vi "Sonde Single Measurement Subvi.vi"(0 "VISAResourceName in":refnum<vi>, 1 "Time Array":dbl[](array[numeric]), 2 "Cumulative Sonde Data":dbl[][](array[numeric]), 3 "Previous time":dbl, 5 "Sonde Data Display":refnum<vi>, 7 "Sonde Graph in":refnum<vi>, 9 "Temp Graph 3":refnum<vi>, 11 "error in (no error)":errorcluster, 12 "Row Cluster Input":T1={"Head\nPressure"=0.0, "Depth"=0.0, "comment "="", "Aux1"=0.0, "Aux2"=0.0, "Aux3\\EC"=0.0, "Sonde Data Cluster"={"Specific\nCond (uS)"=2.0, "Dissolved\nOxygen mg/L"=3.0, "pH"=4.0, "ORP"=5.0, "Temp (deg C)"=26.0, "Salinity"=7.0, "Dissolved\nOxygen (%)"=0.0}, "Cumulative\nVolume (ml)"=100.0} {"Cumulative\nVolume (ml)" format="%#_4g"; "Sonde Data Cluster"."Dissolved\nOxygen (%)" format="%_3g"; "Sonde Data Cluster"."Salinity" format="%_2g"; "Sonde Data Cluster"."Temp (deg C)" format="%_4g"; "Sonde Data Cluster"."ORP" format="%_4g"; "Sonde Data Cluster"."pH" format="%_4g"; "Sonde Data Cluster"."Dissolved\nOxygen mg/L" format="%_4g"; "Sonde Data Cluster"."Specific\nCond (uS)" format="%#_4g"}, 13 "reference 5":refnum<vi>) -> (4 "seconds since 1Jan1904":timestamp, 6 "Cumulative Sonde \nData Out":dbl[][](array[numeric]), 8 "Sample Sheet Data Row Cluster out":T1 {"Cumulative\nVolume (ml)" format="%#_4g"; "Sonde Data Cluster"."Dissolved\nOxygen (%)" format="%_3g"; "Sonde Data Cluster"."Salinity" format="%_2g"; "Sonde Data Cluster"."Temp (deg C)" format="%_4g"; "Sonde Data Cluster"."ORP" format="%_4g"; "Sonde Data Cluster"."pH" format="%_4g"; "Sonde Data Cluster"."Dissolved\nOxygen mg/L" format="%_4g"; "Sonde Data Cluster"."Specific\nCond (uS)" format="%#_4g"}, 10 "output cluster":T2 caption="Cluster" {"Dissolved\nOxygen (%)" format="%_3g"; "Salinity" format="%_2g"; "Temp (deg C)" format="%_4g"; "ORP" format="%_4g"; "pH" format="%_3g"; "Dissolved\nOxygen mg/L" format="%_4g"; "Specific\nCond (uS)" format="%#_4g"}, 14 "time array out":dbl[](array[numeric]), 15 "error out":errorcluster)   [LabVIEW 2016]
uses:
  activeXtest/activeXtest 2015 Folder/sonde cluster.ctl
  activeXtest/activeXtest 2015 Folder/sample data row cluster.ctl
panel:
  in  "Manual Entry Quanta Sonde Com Port":refnum<visa-resource-name>="COM12"
  out "error out 2":errorcluster
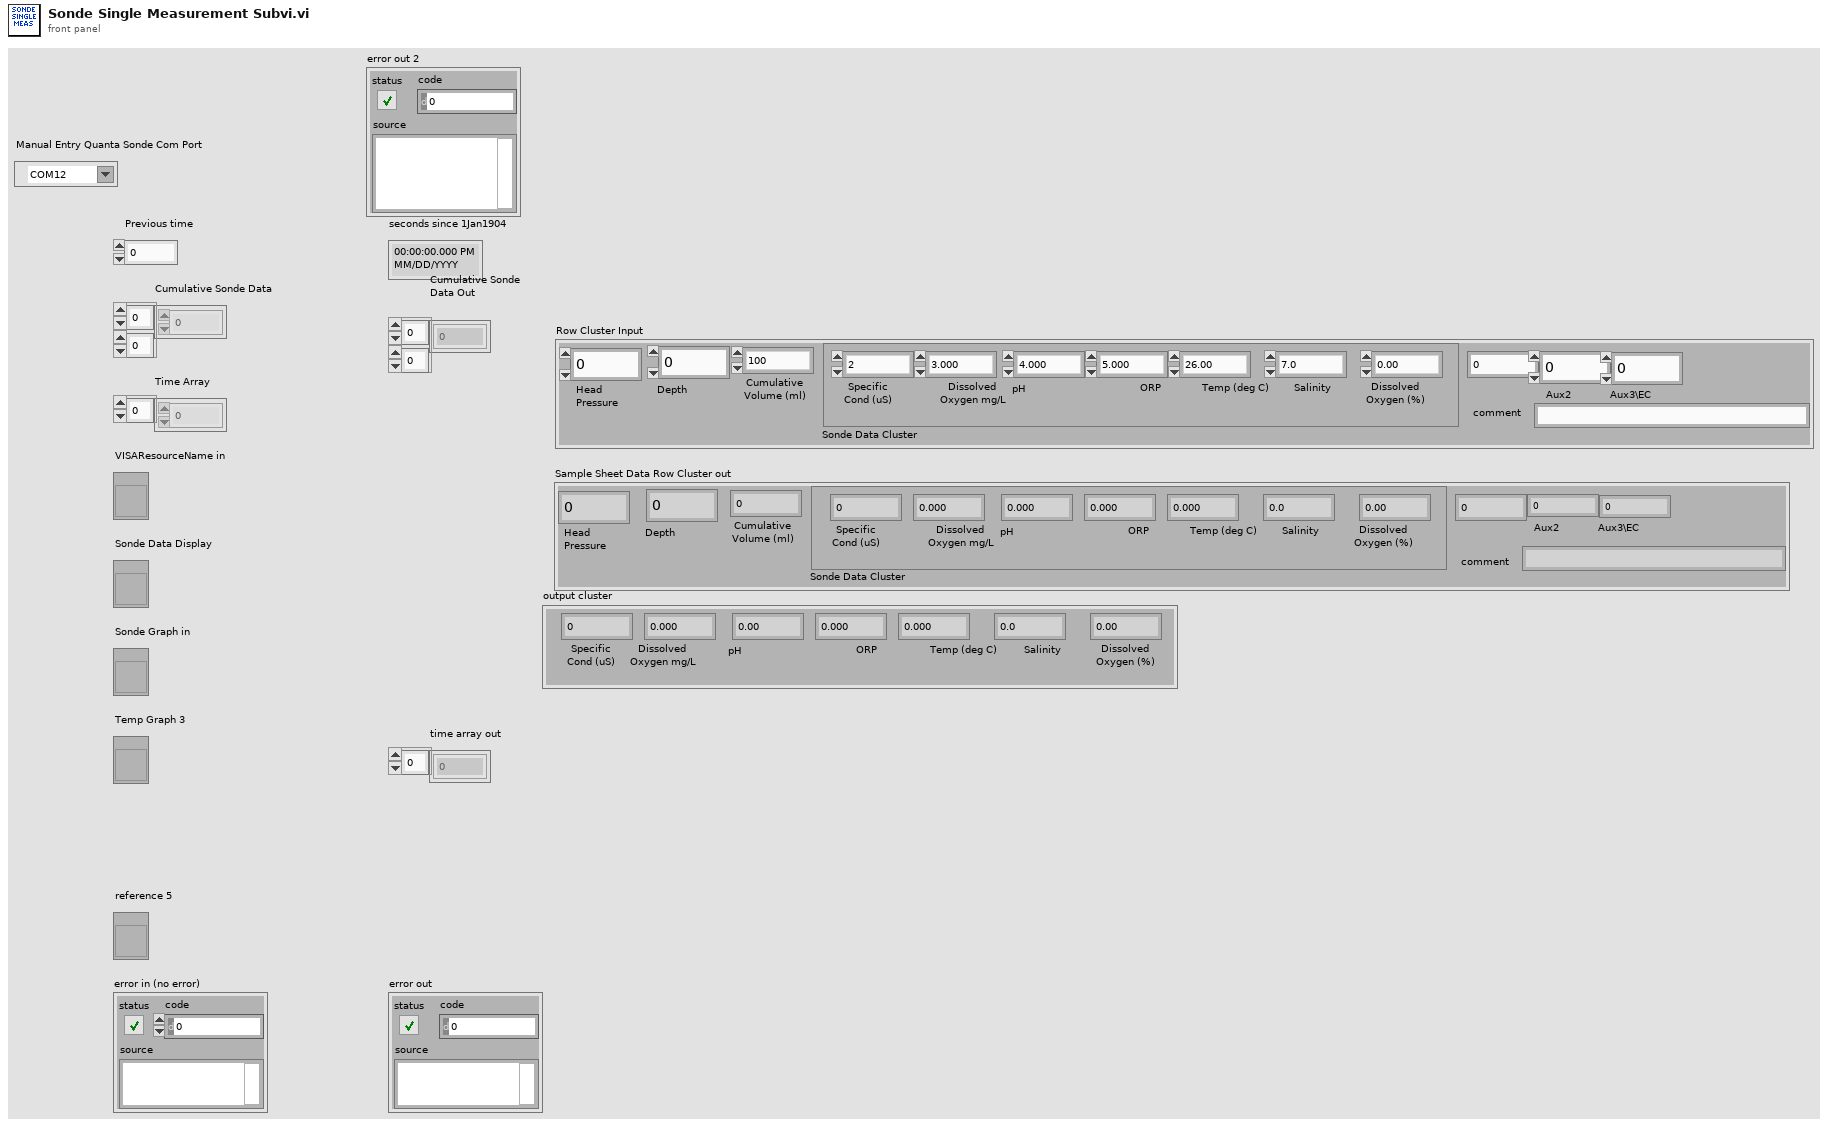
[diagram p1: front panel]
types:
  T1 = typedef "sample data row cluster.ctl" = cluster{"Head\nPressure":dbl, "Depth":dbl, "comment ":string, "Aux1":dbl, "Aux2":dbl, "Aux3\\EC":dbl, "Sonde Data Cluster":T2, "Cumulative\nVolume (ml)":dbl}
  T2 = typedef "sonde cluster.ctl" = cluster{"Specific\nCond (uS)":dbl, "Dissolved\nOxygen mg/L":dbl, "pH":dbl, "ORP":dbl, "Temp (deg C)":dbl, "Salinity":dbl, "Dissolved\nOxygen (%)":dbl}
  T3 = typedef "Sonde Vertical Graph.ctl" = cluster{"pH":T4, "Conductance":T4, "Salinity":T4, "DO % Saturation":T4, "DO mg/L":T4, "ORP":T4}
  T4 = typedef "Vertical Chart.ctl" = cluster{"Y":dbl[], "Y":dbl[]}[]
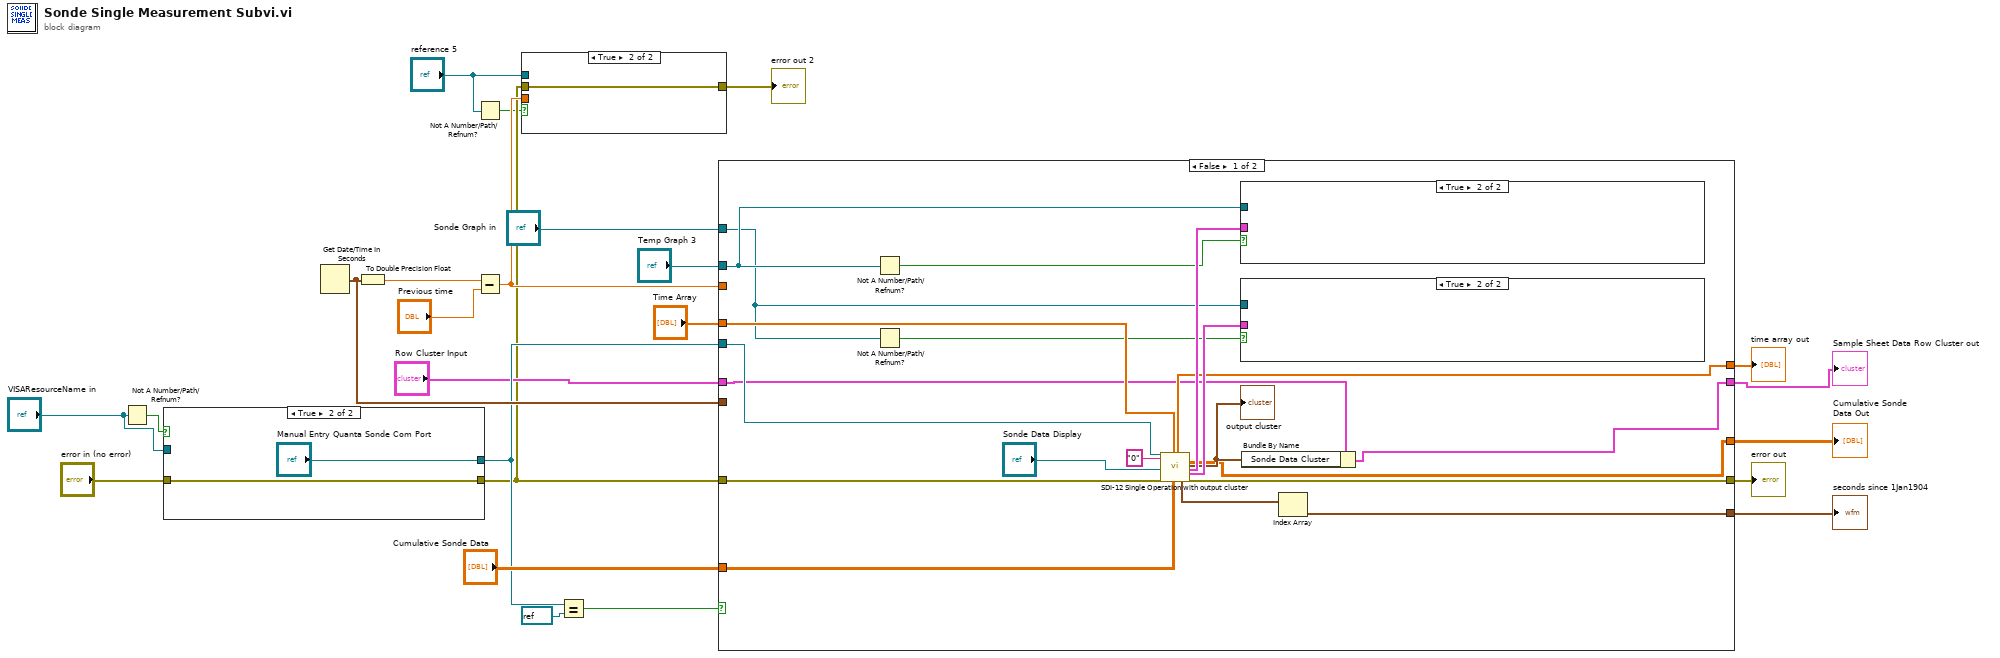
[diagram p0: block diagram]
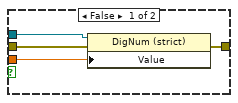
[diagram p2: hidden frame]
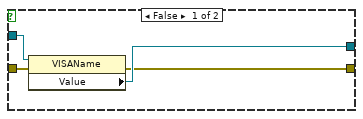
[diagram p3: hidden frame]
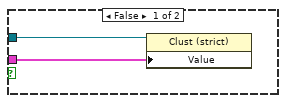
[diagram p4: hidden frame]
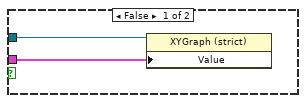
[diagram p5: hidden frame]
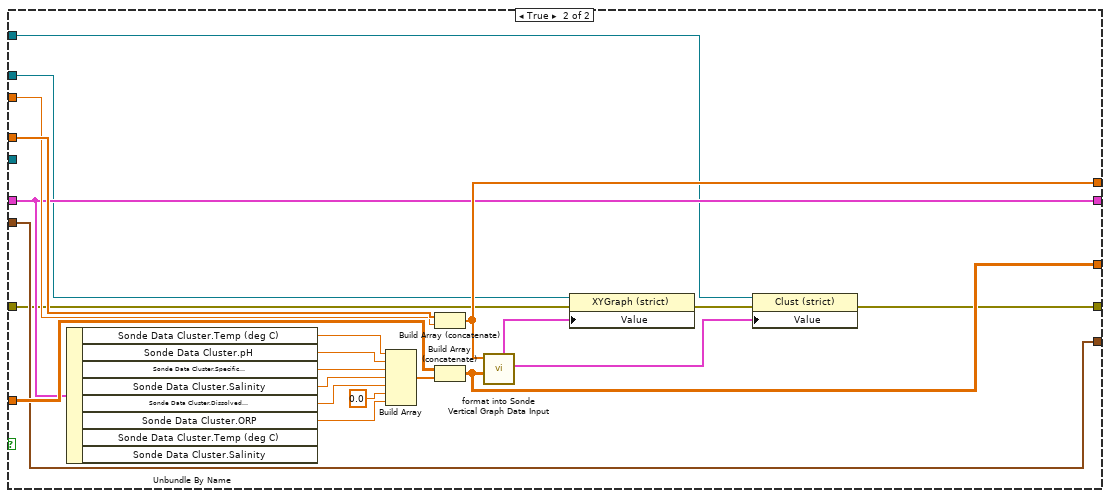
[diagram p6: hidden frame]
diagram:
  n1 = Not A Number/Path/Refnum?(number/path/refnum="VISAResourceName in") -> (NaN/Path/Refnum?=w3:bool)
  n2 = case shown="True" w3 {
    tunnel: [w28 "Manual Entry Quanta Sonde Com Port"] -> w14
    tunnel: "error in (no error)" -> [w27 w30]
    tunnel: [w26 w30] -> w5
    tunnel: "VISAResourceName in" -> [w25 _]
    frame False {
      n3 = property class="VISAName"(reference=w25, error in=w27) -> (error out=w26:errorcluster, "Value"=w28:refnum<visa-resource-name>)  [unwired: 1 out]
    }
    frame True {
    }
  }
  n4 = Get Date/Time In Seconds() -> (seconds since 1Jan1904=w24:timestamp)
  n5 = To Double Precision Float(number=w24) -> (double precision float=w21:dbl)
  n6 = Not A Number/Path/Refnum?(number/path/refnum="reference 5") -> (NaN/Path/Refnum?=w1:bool)
  n7 = Subtract(x=w21, y="Previous time") -> (x-y=w23:dbl)
  n8 = case shown="True" w1 {
    tunnel: w23 -> [w34 _]
    tunnel: "reference 5" -> [w33 _]
    tunnel: [w32 w35] -> w7
    tunnel: w5 -> [w31 w35]
    frame False {
      n9 = property class="DigNum (strict)"(reference=w33, error in=w31, "Value"=w34) -> (error out=w32:errorcluster)  [unwired: 1 out]
    }
    frame True {
    }
  }
  "error out 2" <- w7
  n10 = Equal?(x=w14, y=refnum<visa-resource-name> refnum ("RS232 Port Out")) -> (x = y?=w12:bool)
  n11 = case shown="False" w12 {
    tunnel: w14 -> [w55 _]
    tunnel: [w36 w65] -> w19
    tunnel: w5 -> [w50 w63]
    tunnel: [w49 w62] -> w11
    tunnel: "Time Array" -> [w47 w81]
    tunnel: [w46 w72] -> w16
    tunnel: [w45 w71] -> w17
    tunnel: "Cumulative Sonde Data" -> [w44 w80]
    tunnel: [w42 w66] -> w20
    tunnel: w23 -> [_ w67]
    tunnel: w24 -> [_ w66]
    tunnel: "Sonde Graph in" -> [w39 w60]
    tunnel: "Temp Graph 3" -> [w40 w61]
    tunnel: "Row Cluster Input" -> [w41 w65]
    frame False {
      n12 = Not A Number/Path/Refnum?(number/path/refnum=w40) -> (NaN/Path/Refnum?=w38:bool)
      n13 = Not A Number/Path/Refnum?(number/path/refnum=w39) -> (NaN/Path/Refnum?=w37:bool)
      n14 = call "SDI-12 Single Operation with output cluster.vi"("RS232 Port In"=w55, "Sensor Address In"="0", "Sonde Data Ctl Refnum"="Sonde Data Display", "Error In (No Error)"=w50, "Time Array In"=w47, "Measurement Array In"=w44) -> ("time array out"=w46:dbl[], "Time Array"=w43:timestamp[], "Measurement  array Out"=w45:dbl[][], "output cluster"=w48:T2, "Temperature"=w53:cluster{"Y":dbl[], "Y":dbl[]}[], "Sonde Data Display"=w52:T3, "Error Out"=w49:errorcluster)  [unwired: 12 in, 3 out]
      "output cluster" <- w48
      n15 = case shown="True" w38 {
        tunnel: w53 -> [w59 _]
        tunnel: w40 -> [w58 _]
        frame False {
          n16 = property class="XYGraph (strict)"(reference=w58, "Value"=w59) -> ()  [unwired: 1 in, 2 out]
        }
        frame True {
        }
      }
      n17 = case shown="True" w37 {
        tunnel: w52 -> [w57 _]
        tunnel: w39 -> [w56 _]
        frame False {
          n18 = property class="Clust (strict)"(reference=w56, "Value"=w57) -> ()  [unwired: 1 in, 2 out]
        }
        frame True {
        }
      }
      n19 = Bundle By Name(cluster=w41, "Sonde Data Cluster"=w48) -> (w36:T1)
      n20 = Index Array(array=w43) -> (element=w42:timestamp)  [unwired: 1 in]
    }
    frame True {
      n21 = Unbundle By Name(w65) -> ("Sonde Data Cluster.Temp (deg C)"=w68:dbl, "Sonde Data Cluster.pH"=w79:dbl, "Sonde Data Cluster.Specific\nCond (uS)"=w78:dbl, "Sonde Data Cluster.Salinity"=w77:dbl, "Sonde Data Cluster.Dissolved\nOxygen mg/L"=w76:dbl, "Sonde Data Cluster.ORP"=w75:dbl)  [unwired: 2 out]
      n22 = Build Array(w68, w79, w78, w77, w76, 0.0 ("element"), w75) -> (w73:dbl[])
      n23 = Build Array (concatenate)(w81, w67) -> (w72:dbl[])
      n24 = Build Array (concatenate)(w80, w73) -> (w71:dbl[][])
      n25 = call "format into Sonde Vertical Graph Data Input.vi"("Sonde Measurement Array"=w71, "Time Array"=w72) -> ("Sonde Data Display"=w70:T3, "Temperature"=w69:cluster{"X":dbl[], "Y":dbl[]}[])  [unwired: 8 in]
      n26 = property class="XYGraph (strict)"(reference=w61, error in=w63, "Value"=w69) -> (error out=w64:errorcluster)  [unwired: 1 out]
      n27 = property class="Clust (strict)"(reference=w60, error in=w64, "Value"=w70) -> (error out=w62:errorcluster)  [unwired: 1 out]
    }
  }
  "seconds since 1Jan1904" <- w20
  "Sample Sheet Data Row Cluster out" <- w19
  "Cumulative Sonde \nData Out" <- w17
  "time array out" <- w16
  "error out" <- w11
